vi "test_for_trip.vi"(8 "error in (no error)":errorcluster, 11 "BoardHandle in":T1) -> (0 "error out":errorcluster, 2 "Trip?":bool, 3 "BoardHandle out 3":T1)   [LabVIEW 2020]
uses:
  Program Files/National Instruments/LabVIEW 2018/instr.lib/CAEN PSM/CAEN PSM.lvlib
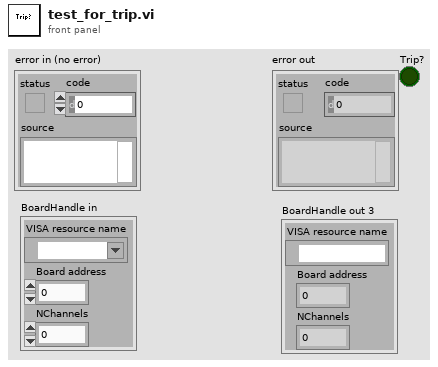
[diagram p1: front panel]
types:
  T1 = cluster{"VISA resource name":refnum<visa-resource-name>, "Board address":u8, "NChannels":u8}
  T2 = cluster{"ON":bool, "RUP":bool, "RDW":bool, "OVC":bool, "OVV":bool, "UNV":bool, "MAXV":bool, "TRIP":bool, "OVP":bool, "OVT":bool, "DIS":bool, "KILL":bool, "ILK":bool, "NOCAL":bool}[]
  T3 = typedef "CAEN PSM.lvlib/BoardHandle.ctl" = cluster{"VISA resource name":refnum<visa-resource-name>, "Board address":u8, "NChannels":u8}
  T4 = cluster{"ON":bool, "RUP":bool, "RDW":bool, "OVC":bool, "OVV":bool, "UNV":bool, "MAXV":bool, "TRIP":bool, "OVP":bool, "OVT":bool, "DIS":bool, "KILL":bool, "ILK":bool, "NOCAL":bool}
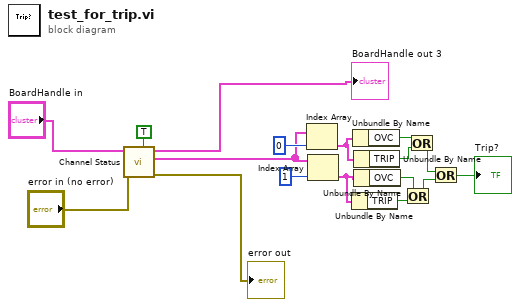
[diagram p0: block diagram]
diagram:
  n1 = call "Channel Status.vi"("All Channels (T)"=TRUE, "error in (no error)"="error in (no error)", "BoardHandle"="BoardHandle in") -> ("error out"=→"error out":errorcluster, "Channel Status Array"=w14:T2, "BoardHandle out"=→"BoardHandle out 3":T3)  [unwired: 6 in]
  n2 = Index Array(array=w14, index=0) -> (element=w9:T4)
  n3 = Index Array(array=w14, index=1) -> (element=w13:T4)
  n4 = Unbundle By Name(w13) -> ("TRIP"=w11:bool)
  n5 = Unbundle By Name(w9) -> ("OVC"=w8:bool)
  n6 = Unbundle By Name(w9) -> ("TRIP"=w7:bool)
  n7 = Unbundle By Name(w13) -> ("OVC"=w12:bool)
  n8 = Or(x=w12, y=w11) -> (x .or. y?=w10:bool)
  n9 = Or(x=w8, y=w7) -> (x .or. y?=w6:bool)
  n10 = Or(x=w6, y=w10) -> (x .or. y?=→"Trip?":bool)
